vi "LoadControlValues.vi"(8 "error in":errorcluster, 11 "ControlValues in":refnum<class "ControlValues.lvclass">) -> (0 "error out":errorcluster, 3 "ControlValues out":refnum<class "ControlValues.lvclass">)   [LabVIEW 2014, in "ControlValues.lvclass"]
uses:
  ControlValues.lvclass
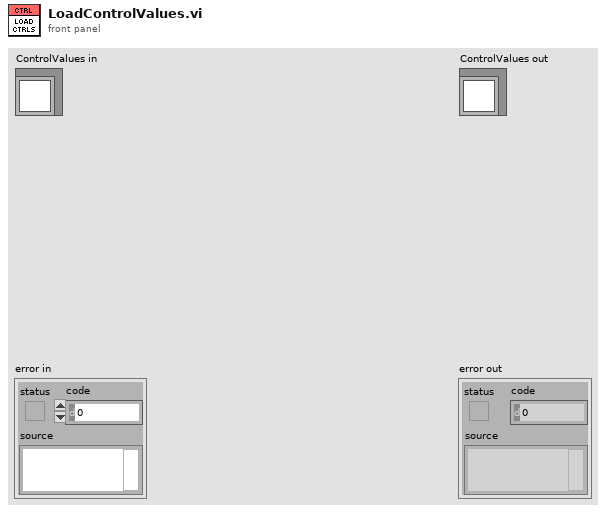
[diagram p1: front panel]
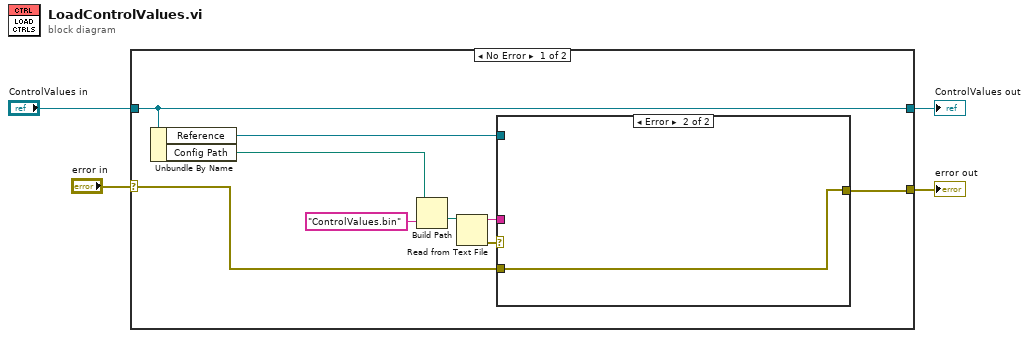
[diagram p0: block diagram]
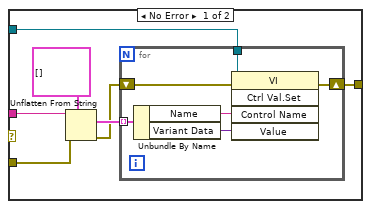
[diagram p2: hidden frame]
diagram:
  n1 = case shown="No Error" "error in" {
    selector: "error in" -> [w7 w29]
    tunnel: [w8 w29] -> w3
    tunnel: [w12 w28] -> w1
    tunnel: "ControlValues in" -> [w12 w28]
    frame No Error {
      n2 = Unbundle By Name(w12) -> ("Reference"=w11:refnum<vi>, "Config Path"=w5:path)
      n3 = Build Path(base path=w5, name or relative path="ControlValues.bin") -> (appended path=w9:path)
      n4 = Read from Text File(file (use dialog)=w9) -> (text=w13:string, error out=w6:errorcluster)  [unwired: 3 in, 2 out]
      n5 = case shown="Error" w6 {
        tunnel: w13 -> [w20 _]
        tunnel: w11 -> [w17 _]
        tunnel: [w15 w27] -> w8
        tunnel: w7 -> [w14 w27]
        frame No Error {
          n6 = Unflatten From String(type=cluster{"Name":string, "Variant Data":variant}[] [] ("Control Value:Get All"), binary string=w20, error in (no error)=w14) -> (value=w18:cluster{"Name":string, "Variant Data":variant}[], error out=w16:errorcluster)  [unwired: 2 in, 1 out]
          n7 = for {
            tunnel: w18 -> [w26] mode=indexing
            tunnel: w17 -> [w23]
            shift-right: [w21] -> w15
            shift-left: w16 -> [w22]
            n8 = Unbundle By Name(w26) -> ("Name"=w25:string, "Variant Data"=w24:variant)
            n9 = invoke class="VI" method="Ctrl Val.Set"(reference=w23, error in=w22, "Control Name"=w25, "Value"=w24) -> (error out=w21:errorcluster)  [unwired: 1 in, 4 out]
          }
        }
        frame Error {
        }
      }
    }
    frame Error {
    }
  }
  "error out" <- w3
  "ControlValues out" <- w1
